vi "Create Evaluations.vi"(8 "error in (no error)":errorcluster, 11 "IEvaluation in":refnum<class "DC_IDD.lvclass">) -> (0 "error out":errorcluster, 2 "Evaluations Out":T1[](array[typedef]) {"Low Limit" format="%#_13g"; "SI Scaling" items=["femto"=-15, "pico"=-12, "nano"=-9, "micro"=-6, "milli"=-3, "percent"=-2, ""=0, "kilo"=3, "mega"=6, "giga"=9, "tera"=12]}, 3 "IEvaluation out":refnum<class "DC_IDD.lvclass">)   [LabVIEW 2016, in "SeqAuto Evaluations.lvlib" / "DC_IDD.lvclass"]
uses:
  DC_IDD.lvclass
  C:/Sequence Automation/Plugins/SeqAuto IEvaluation.lvlibp/SeqAuto IEvaluation.lvclass
  Plugins/TestStand API Tools (TSAT).lvlibp/Evaluation Actions/Includes/Controls/TSAT Evaluation.ctl
  Plugins/TestStand API Tools (TSAT).lvlibp/Evaluation Actions/Includes/Controls/TSAT Eval SI Unit Scaling.ctl
  Plugins/TestStand API Tools (TSAT).lvlibp/Evaluation Actions/Includes/Controls/TSAT Evaluation Type.ctl
  DC_IDD.lvclass/DC_IDD.ctl
  Plugins/SeqAuto IEvaluation.lvlibp/Read Measurement Name.vi
  Plugins/TestStand API Tools (TSAT).lvlibp/Evaluation Actions/TSAT Evaluation Actions.lvlib
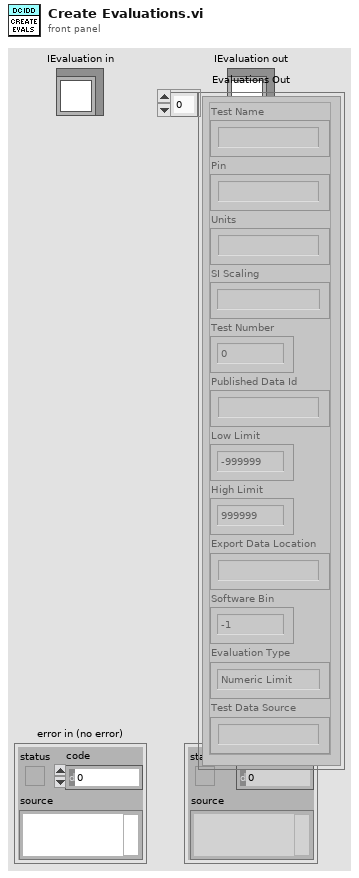
[diagram p1: front panel]
types:
  T1 = typedef "TestStand API Tools (TSAT).lvlibp/TSAT Evaluation Actions.lvlib/TSAT Evaluation.ctl" = cluster{"Test Name":string, "Pin":string, "Units":string, "SI Scaling":T2, "Test Number":i32, "Published Data Id":string, "Low Limit":dbl, "High Limit":dbl, "Export Data Location":string, "Software Bin":i64, "Evaluation Type":T3, "Test Data Source":string}
  T2 = typedef "TestStand API Tools (TSAT).lvlibp/TSAT Evaluation Actions.lvlib/TSAT Eval SI Unit Scaling.ctl" = i16
  T3 = typedef "TestStand API Tools (TSAT).lvlibp/TSAT Evaluation Actions.lvlib/TSAT Evaluation Type.ctl" = enum16{"Numeric Limit", "Pass/Fail", "None"}
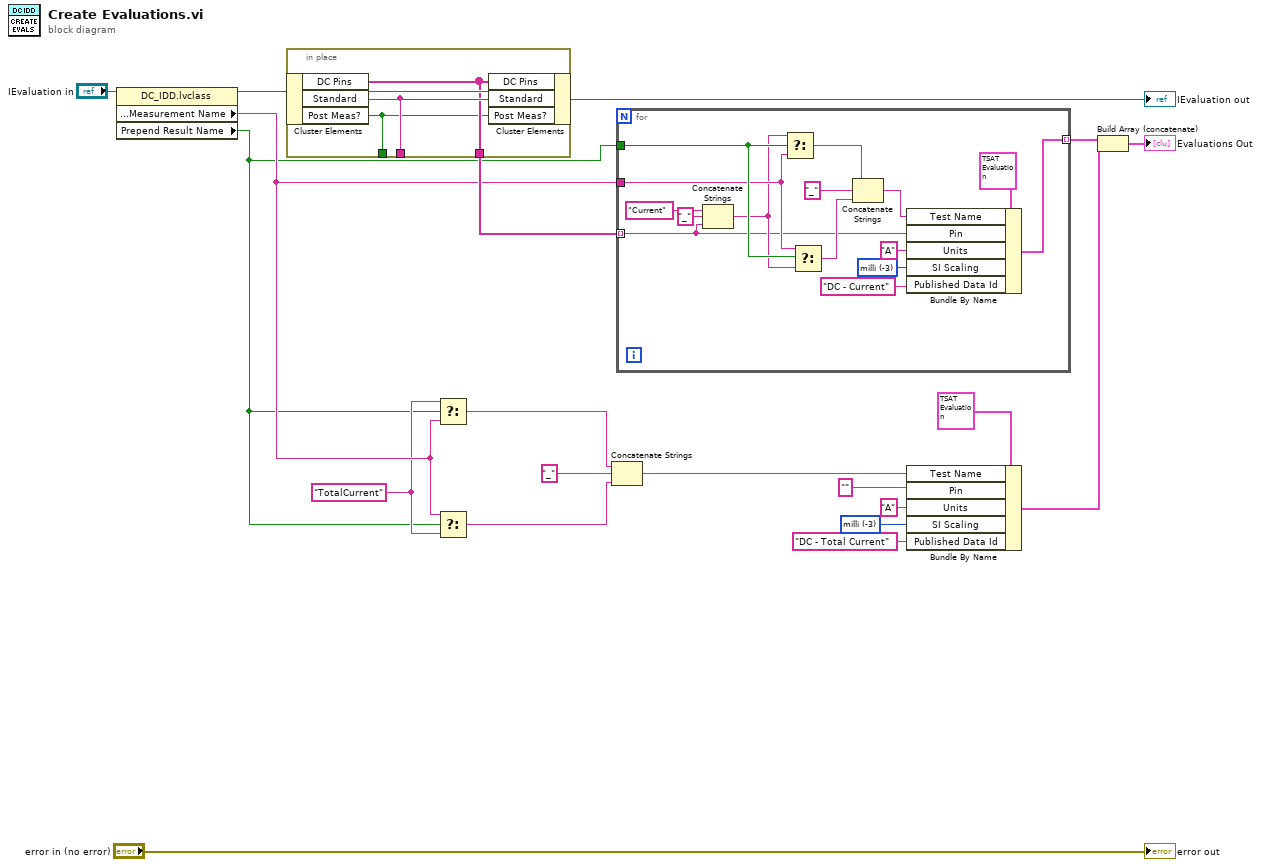
[diagram p0: block diagram]
diagram:
  w11 = T2 -3 items=["femto"=-15, "pico"=-12, "nano"=-9, "micro"=-6, "milli"=-3, "percent"=-2, ""=0, "kilo"=3, "mega"=6, "giga"=9, "tera"=12] ("SI Scaling")
  w3 = "TotalCurrent" ("Test Name")
  n1 = property class="DC_IDD.lvclass"(reference="IEvaluation in") -> (reference out=w18:refnum<class "DC_IDD.lvclass">, "Protected Methods:Measurement Name"=w4:string, "Prepend Result Name"=w1:bool)  [unwired: 1 in, 1 out]
  n2 = in-place {
    in-place-border: [w23] -> w16
    in-place-border: [w22] -> _
    in-place-border: [w21] -> _
    n3 = in-place-cluster #1(w18) -> ("DC Pins"=w23:string[], "Standard"=w22:string, "Post Meas?"=w21:bool)
    n4 = in-place-cluster #1("DC Pins"=w23, "Standard"=w22, "Post Meas?"=w21) -> (→"IEvaluation out":refnum<class "DC_IDD.lvclass">)
  }
  n5 = Select(t=w3, s=w1, f=w4) -> (s? t:f=w5:string)
  n6 = Select(t=w4, s=w1, f=w3) -> (s? t:f=w2:string)
  n7 = Concatenate Strings(w5, "_" ("string"), w2) -> (w7:string)
  n8 = for {
    tunnel: [w37] -> w15 mode=indexing
    tunnel: w4 -> [w29]
    tunnel: w16 -> [w24] mode=indexing
    tunnel: w1 -> [w31]
    w35 = T2 -3 items=["femto"=-15, "pico"=-12, "nano"=-9, "micro"=-6, "milli"=-3, "percent"=-2, ""=0, "kilo"=3, "mega"=6, "giga"=9, "tera"=12] ("SI Scaling")
    n9 = Concatenate Strings("Current" ("string"), "_" ("string"), w24) -> (w27:string)
    n10 = Select(t=w27, s=w31, f=w29) -> (s? t:f=w28:string)
    n11 = Select(t=w29, s=w31, f=w27) -> (s? t:f=w30:string)
    n12 = Concatenate Strings(w28, "_" ("string"), w30) -> (w36:string)
    n13 = Bundle By Name(cluster=T1 {"Test Name"="", "Pin"="", "Units"="", "SI Scaling"=0, "Test Number"=0, "Published Data Id"="", "Low Limit"=-999999.0, "High Limit"=999999.0, "Export Data Location"="", "Software Bin"=-1, "Evaluation Type"=enum."Numeric Limit", "Test Data Source"=""} ("Evaluation"), "Test Name"=w36, "Pin"=w24, "Units"="A", "SI Scaling"=w35, "Published Data Id"="DC - Current") -> (w37:T1)
  }
  n14 = Bundle By Name(cluster=T1 {"Test Name"="", "Pin"="", "Units"="", "SI Scaling"=0, "Test Number"=0, "Published Data Id"="", "Low Limit"=-999999.0, "High Limit"=999999.0, "Export Data Location"="", "Software Bin"=-1, "Evaluation Type"=enum."Numeric Limit", "Test Data Source"=""} ("Evaluation"), "Test Name"=w7, "Pin"="", "Units"="A", "SI Scaling"=w11, "Published Data Id"="DC - Total Current") -> (w8:T1)
  n15 = Build Array (concatenate)(w15, w8) -> (→"Evaluations Out":T1[])
  "error out" <- "error in (no error)"
